vi "read_byte_to_queue.vi"(7 "Queue in":refnum<queue>, 8 "error in (no error)":errorcluster, 11 "VISA resource name in":refnum<visa-resource-name>) -> (0 "error out":errorcluster, 3 "VISA Refnum out":refnum<visa-resource-name>)   [LabVIEW 2024]
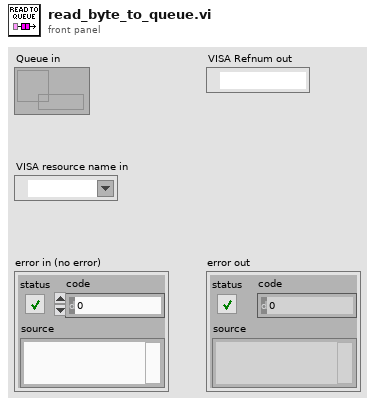
[diagram p1: front panel]
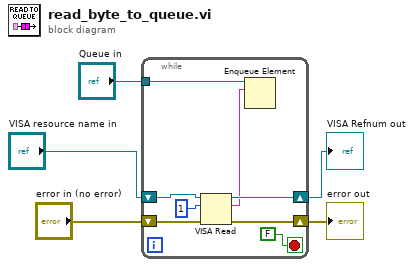
[diagram p0: block diagram]
diagram:
  n1 = while {
    shift-right: [w13] -> w4
    shift-left: "VISA resource name in" -> [w12]
    shift-right: [w8] -> w3
    shift-left: "error in (no error)" -> [w11]
    tunnel: "Queue in" -> [w7]
    stop <- FALSE stop-if-true
    n2 = VISA Read(VISA resource name=w12, byte count=u32 1, error in (no error)=w11) -> (VISA resource name out=w13:refnum<visa-resource-name>, read buffer=w9:string, error out=w8:errorcluster)  [unwired: 1 out]
    n3 = Enqueue Element(queue=w7, element=w9) -> ()  [unwired: 2 in, 3 out]
  }
  "VISA Refnum out" <- w4
  "error out" <- w3
